vi "Write fs_px.vi"(8 "error in (no error)":errorcluster, 10 "fs/px":dbl[unit], 11 "Analyze Parameter Temporal Calibration in":refnum<class "Analyze Parameter Temporal Calibration.lvclass">) -> (0 "error out":errorcluster, 3 "Analyze Parameter Temporal Calibration out":refnum<class "Analyze Parameter Temporal Calibration.lvclass">)   [LabVIEW 2014, in "Analyze Parameter Temporal Calibration.lvclass"]
uses:
  Analyze Parameter Temporal Calibration.lvclass
  Analyze Parameter Temporal Calibration.lvclass/Analyze Parameter Temporal Calibration.ctl
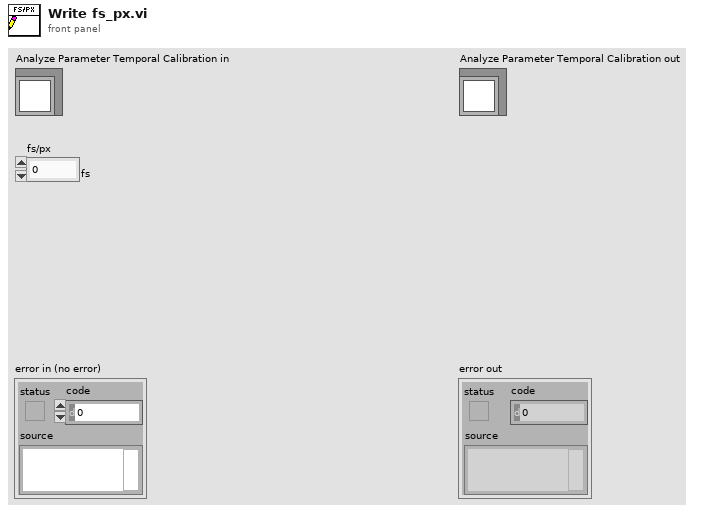
[diagram p1: front panel]
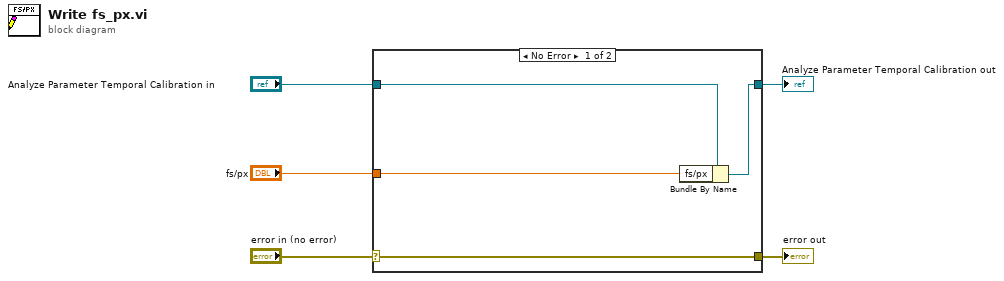
[diagram p0: block diagram]
diagram:
  n1 = case shown="No Error" "error in (no error)" {
    selector: "error in (no error)" -> [w9 w10]
    tunnel: [w9 w10] -> w4
    tunnel: [w7 w11] -> w2
    tunnel: "Analyze Parameter Temporal Calibration in" -> [w8 w11]
    tunnel: "fs/px" -> [w6 _]
    frame No Error {
      n2 = Bundle By Name(cluster=w8, "fs/px"=w6) -> (w7:refnum<class "Analyze Parameter Temporal Calibration.lvclass">)
    }
    frame Error {
    }
  }
  "error out" <- w4
  "Analyze Parameter Temporal Calibration out" <- w2
